vi "Query Info Log.vi"(6 "timeout (ms)":i32=5000, 8 "error in":errorcluster, 10 "query_all":bool, 11 "gRPC ID in":T1) -> (0 "error out":errorcluster, 2 "Info":string, 3 "gRPC ID out":T1)   [LabVIEW 2021, in "CIFManagerClientWrapper.lvlib"]
uses:
  CIFManagerClientWrapper.lvlib
  <vilib>/gRPC/LabVIEW gRPC Library/Shared/grpcId.ctl
  CIF_Manager_client/RPC Messages/cif_manager_QueryInfoRequest.ctl
  CIF_Manager_client/RPC Messages/cif_manager_QuerySettings.ctl
  CIF_Manager_client/CIF_Manager_client.lvlib
  <vilib>/gRPC/LabVIEW gRPC Library/grpc-lvsupport-release.lvlib
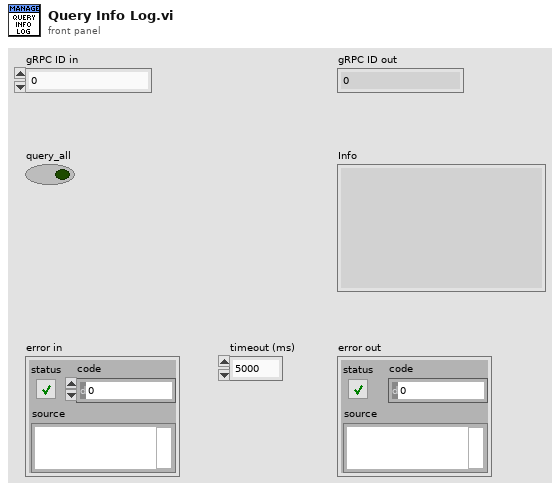
[diagram p1: front panel]
types:
  T1 = typedef "grpc-lvsupport-release.lvlib/grpcId.ctl" = u64
  T2 = typedef "CIF_Manager_client.lvlib/cif_manager_QueryInfoRequest.ctl" = cluster{"query_settings":T3}
  T3 = typedef "CIF_Manager_client.lvlib/cif_manager_QuerySettings.ctl" = cluster{"query_all":bool}
  T4 = typedef "CIF_Manager_client.lvlib/cif_manager_QueryInfoResponse.ctl" = cluster{"file_data":T5}
  T5 = typedef "CIF_Manager_client.lvlib/cif_manager_FileData.ctl" = cluster{"data":string}
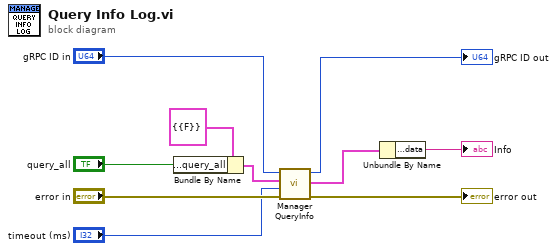
[diagram p0: block diagram]
diagram:
  n1 = Bundle By Name(cluster=T2 {"query_settings"={"query_all"=FALSE}} ("Request Data"), "query_settings.query_all"="query_all") -> (w1:T2)
  n2 = call "Manager QueryInfo.vi"("error in"="error in", "timeout (ms)"="timeout (ms)", "Request Data"=w1, "gRPC ID"="gRPC ID in") -> ("error out"=→"error out":errorcluster, "Response Data"=w5:T4, "gRPC ID out"=→"gRPC ID out":T1)  [unwired: 5 in]
  n3 = Unbundle By Name(w5) -> ("file_data.data"=→"Info":string)
